vi "Check If Line Exists.vi"(8 "error in (no error)":errorcluster, 10 "Name to locate":string, 11 "Modbus Slave configuration in":refnum<class "Modbus Module configuration.lvclass">) -> (0 "error out":errorcluster, 1 "Index":i32, 2 "Line out":T1, 3 "Modbus Slave configuration out":refnum<class "Modbus Module configuration.lvclass">, 5 "Found?":bool)   [LabVIEW 2013, in "Modbus Module configuration.lvclass"]
uses:
  Modbus Module configuration.lvclass
  Line.ctl
  module channel/Modbus Module Channel.lvclass
  Modbus Module configuration.lvclass/Modbus Module configuration.ctl
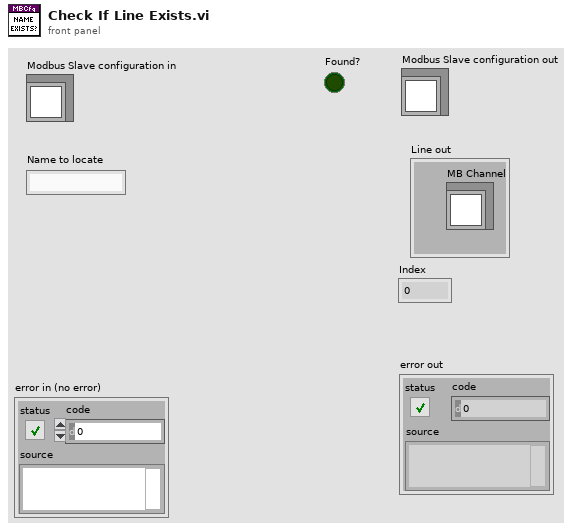
[diagram p1: front panel]
types:
  T1 = typedef "Modbus Module configuration.lvclass/Line.ctl" = cluster{"MB Channel":refnum<class "Modbus Module Channel.lvclass">}
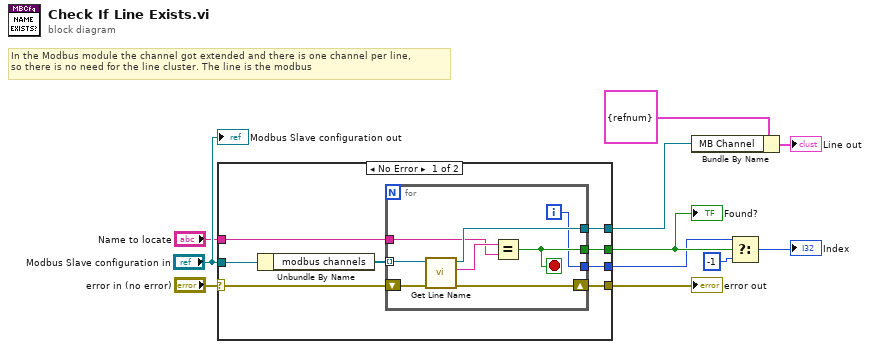
[diagram p0: block diagram]
diagram:
  # "In the Modbus module the channel got extended and there is one channel per line, \nso there is no need for the line cluster. The line is the modbus"
  n1 = case shown="No Error" "error in (no error)" {
    selector: "error in (no error)" -> [w13 w28]
    tunnel: [w12 w28] -> w10
    tunnel: "Modbus Slave configuration in" -> [w19 _]
    tunnel: [w17 _] -> w2
    tunnel: "Name to locate" -> [w16 _]
    tunnel: [w15 _] -> w7
    tunnel: [w14 _] -> w6
    frame No Error {
      n2 = Unbundle By Name(w19) -> ("modbus channels"=w18:refnum<class "Modbus Module Channel.lvclass">[])
      n3 = for {
        tunnel: w18 -> [w27] mode=indexing
        tunnel: [w26] -> w17
        tunnel: w16 -> [w24]
        tunnel: [w23] -> w15
        tunnel: [w22] -> w14
        shift-right: [w20] -> w12
        shift-left: w13 -> [w21]
        i -> [w22]
        stop <- w23 stop-if-true
        n4 = call "Get Line Name.vi"("error in"=w21, "MB Channel"=w27) -> ("error out"=w20:errorcluster, "Name"=w25:string, "MB Channel"=w26:refnum<class "Modbus Module Channel.lvclass">)  [unwired: 7 in]
        n5 = Equal?(x=w25, y=w24) -> (x = y?=w23:bool)
      }
    }
    frame Error {
    }
  }
  "Found?" <- w7
  "error out" <- w10
  n6 = Bundle By Name(cluster=T1 {"MB Channel"=refnum} ("Line out"), "MB Channel"=w2) -> (→"Line out":T1)
  n7 = Select(t=w6, s=w7, f=-1) -> (s? t:f=→"Index":i32)
  "Modbus Slave configuration out" <- "Modbus Slave configuration in"
